vi "Init State Control.vi"(8 "error in (no error)":errorcluster, 11 "Sequence in":refnum<class "Sequence.lvclass">) -> (0 "error out":errorcluster, 3 "Sequence out":refnum<class "Sequence.lvclass">)   [LabVIEW 2020, in "VolatusSeq.lvlib" / "Sequence.lvclass"]
uses:
  Sequence.lvclass
  Sequence Time.ctl
  State Control.ctl
  Sequence.lvclass/Sequence.ctl
  VolatusSeq.lvlib
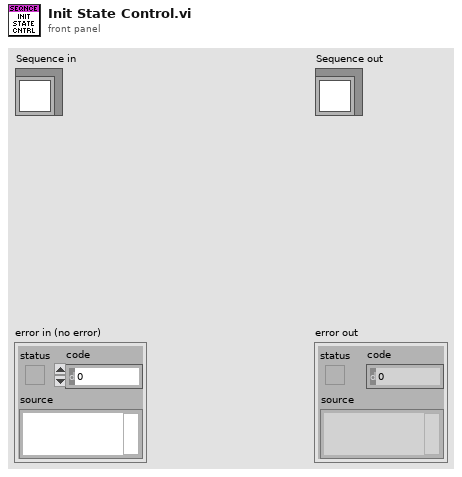
[diagram p1: front panel]
types:
  T1 = typedef "VolatusSeq.lvlib/State Control.ctl" = cluster{"State":refnum<notifier>, "Time":refnum<notifier>, "Request State":refnum<notifier>, "Abort":refnum<notifier>, "Reset":refnum<notifier>, "Close":refnum<notifier>}
  T2 = typedef "VolatusSeq.lvlib/Sequence Time.ctl" = cluster{"Abort":bool, "Seq Time":dbl, "State Time":dbl, "Wall Time":dbl}
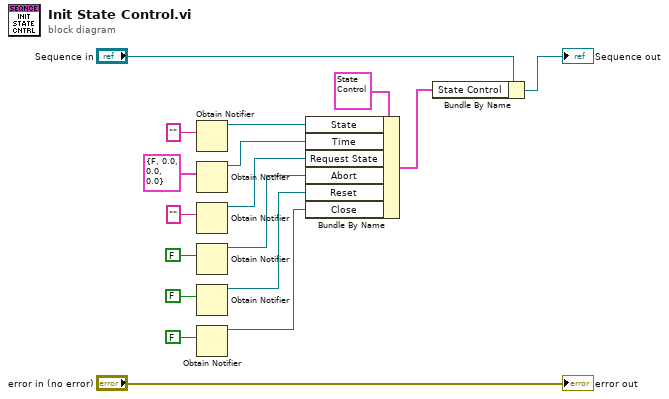
[diagram p0: block diagram]
diagram:
  n1 = Obtain Notifier(notification data type="") -> (notifier out=w12:refnum<notifier>)  [unwired: 3 in, 2 out]
  n2 = Obtain Notifier(notification data type=T2 {"Abort"=FALSE, "Seq Time"=0.0, "State Time"=0.0, "Wall Time"=0.0} ("Sequence State")) -> (notifier out=w11:refnum<notifier>)  [unwired: 3 in, 2 out]
  n3 = Obtain Notifier(notification data type="") -> (notifier out=w7:refnum<notifier>)  [unwired: 3 in, 2 out]
  n4 = Obtain Notifier(notification data type=FALSE) -> (notifier out=w5:refnum<notifier>)  [unwired: 3 in, 2 out]
  n5 = Obtain Notifier(notification data type=FALSE) -> (notifier out=w3:refnum<notifier>)  [unwired: 3 in, 2 out]
  n6 = Obtain Notifier(notification data type=FALSE) -> (notifier out=w1:refnum<notifier>)  [unwired: 3 in, 2 out]
  n7 = Bundle By Name(cluster=T1 {"State"=refnum, "Time"=refnum, "Request State"=refnum, "Abort"=refnum, "Reset"=refnum, "Close"=refnum} ("Control"), "State"=w12, "Time"=w11, "Request State"=w7, "Abort"=w5, "Reset"=w3, "Close"=w1) -> (w9:T1)
  n8 = Bundle By Name(cluster="Sequence in", "State Control"=w9) -> (→"Sequence out":refnum<class "Sequence.lvclass">)
  "error out" <- "error in (no error)"
